vi "Name.vi"(8 "error in (no error)":errorcluster, 11 "Channel Buffer DBL in":refnum<class "Channel Buffer DBL.lvclass">) -> (0 "error out":errorcluster, 2 "Name":string, 3 "Channel Buffer DBL out":refnum<class "Channel Buffer DBL.lvclass">)   [LabVIEW 2020, in "VolatusHistorian.lvlib" / "Channel Buffer DBL.lvclass"]
uses:
  Channel Buffer DBL.lvclass
  Channel Buffer DBL.lvclass/Channel Buffer DBL.ctl
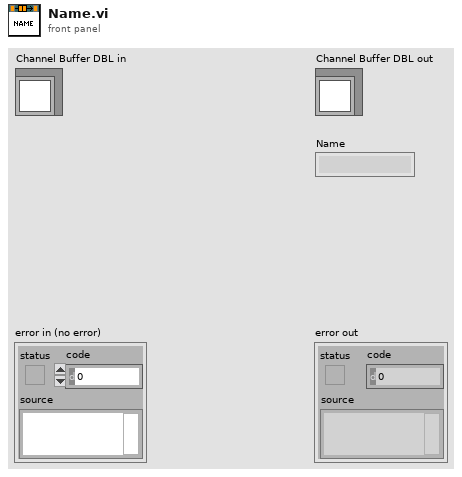
[diagram p1: front panel]
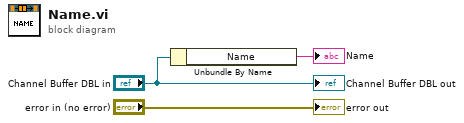
[diagram p0: block diagram]
diagram:
  n1 = Unbundle By Name("Channel Buffer DBL in") -> ("Name"=→"Name":string)
  "error out" <- "error in (no error)"
  "Channel Buffer DBL out" <- "Channel Buffer DBL in"
